vi "Configure PID Cutback Parameters.vi"(0 "VISA resource name":refnum<visa-resource-name>, 1 "Unit Address (1)":u8=1 min=1 max=254, 9 "Cutback High (0)":sgl min=0 max=9999, 11 "error in (no error)":errorcluster, 12 "Cutback Low (0)":sgl min=0 max=9999) -> (4 "VISA resource name out":refnum<visa-resource-name>, 15 "error out":errorcluster)   [LabVIEW 2010, in "Eurotherm 32xx Series.lvlib"]
doc: "This VI sets PID Cutback Parameters.\n\nHigh and low cutback parameters are used to reduce overshoot and undershoot for large step changes in the process."
uses:
  <instrlib>/Eurotherm 32xx Series/Eurotherm 32xx Series.lvlib
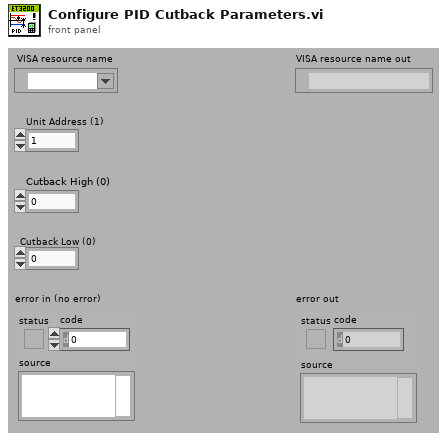
[diagram p1: front panel]
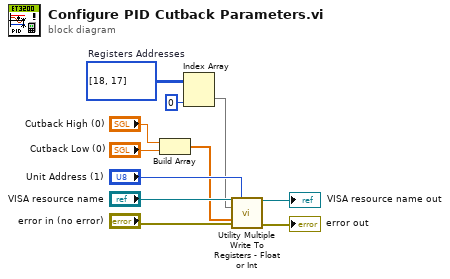
[diagram p0: block diagram]
diagram:
  w11 = u16[][] [[18], [17]]  # Registers Addresses
  n1 = Build Array("Cutback High (0)", "Cutback Low (0)") -> (w2:sgl[])
  n2 = Index Array(array=w11, index (col)=0 ("Number of PID (1)")) -> (element=w3:u16[])  [unwired: 1 in]
  n3 = call <instrlib>:"Utility Multiple Write To Registers - Float or Int.vi"("VISA resource name"="VISA resource name", "Unit Address (1)"="Unit Address (1)", "Registers Addresses (0)"=w3, "Data (0)"=w2, "error in (no error)"="error in (no error)") -> ("VISA resource name out"=→"VISA resource name out":refnum<visa-resource-name>, "error out"=→"error out":errorcluster)  [unwired: 9 in]
